vi "GasflascheInListeFinden.vi"(10 "Gasflasche":T2 {"Ablaufdatum" format="%<%d.%m.%Y>T"}, 11 "GasflaschenListe":T1[](array[typedef]) {"Gasflasche"."Ablaufdatum" format="%<%d.%m.%Y>T"; "Komponenten"."Konzentration IST" format="%#.4f"; "Komponenten"."Genauigkeit" format="%#.1f"}) -> (1 "gefunden":bool, 2 "Index":i32, 3 "GasflaschenListe out":T1[](array[typedef]) {"Gasflasche"."Ablaufdatum" format="%<%d.%m.%Y>T"; "Komponenten"."Konzentration IST" format="%#.4f"; "Komponenten"."Genauigkeit" format="%#.1f"})   [LabVIEW 2020, in "System Einstellungen V2.lvlib"]
uses:
  System Einstellungen V2.lvlib
  Gasflasche.ctl
  Gasflasche gesamt.ctl
  Traegergas.ctl
  Gasflaschenkomponente.ctl
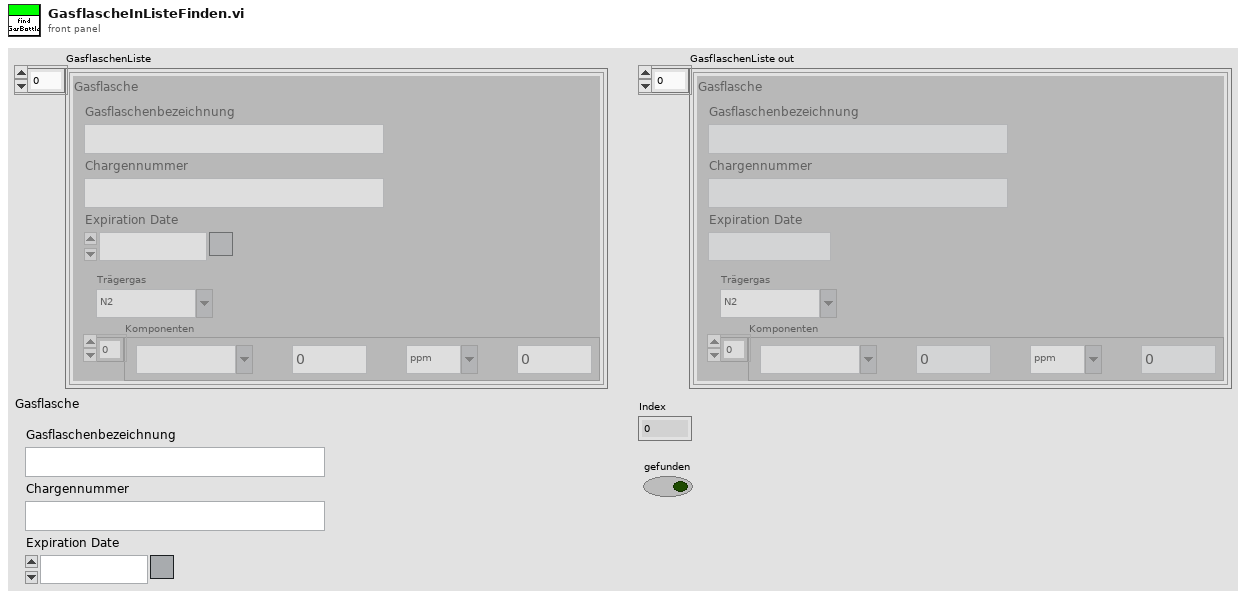
[diagram p1: front panel]
types:
  T1 = typedef "System Einstellungen V2.lvlib/Gasflasche gesamt.ctl" = cluster{"Gasflasche":T2, "Trägergas":T3, "Komponenten":T4[]}
  T2 = typedef "System Einstellungen V2.lvlib/Gasflasche.ctl" = cluster{"Gasname für die Auswahl":string, "Chargennummer":string, "Ablaufdatum":timestamp}
  T3 = typedef "System Einstellungen V2.lvlib/Traegergas.ctl" = string
  T4 = typedef "System Einstellungen V2.lvlib/Gasflaschenkomponente.ctl" = cluster{"Gasauswahl":string, "Konzentration IST":dbl, "Einheit":string, "Genauigkeit":dbl}
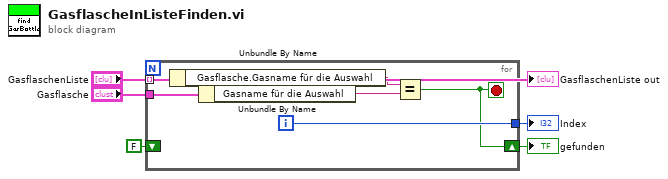
[diagram p0: block diagram]
diagram:
  n1 = for {
    tunnel: "Gasflasche" -> [w10]
    tunnel: "GasflaschenListe" -> [w11] mode=indexing
    tunnel: [w7] -> w4
    shift-right: [w6] -> w1
    shift-left: FALSE -> [_]
    i -> [w7]
    stop <- w6 stop-if-true
    n2 = Unbundle By Name(w11) -> ("Gasflasche.Gasname für die Auswahl"=w9:string)
    n3 = Unbundle By Name(w10) -> ("Gasname für die Auswahl"=w8:string)
    n4 = Equal?(x=w9, y=w8) -> (x = y?=w6:bool)
  }
  "Index" <- w4
  "gefunden" <- w1
  "GasflaschenListe out" <- "GasflaschenListe"
